vi "Update State.vi"(8 "error in (no error)":errorcluster, 11 "MF3 in":refnum<class "MF3.lvclass">) -> (0 "error out":errorcluster, 2 "fail?":bool, 3 "MF3 out":refnum<class "MF3.lvclass">)   [LabVIEW 2011, in "MF3.lvclass"]
uses:
  MF3.lvclass
  Controls/Motor Names.ctl
  MF3.lvclass/MF3.ctl
  <vilib>/Utility/error.llb/Error Cluster From Error Code.vi
  <vilib>/rvi/errors/niLvFpgaAdjustHostInterfaceError.vi
  <vilib>/rvi/interface/nirviReadWriteControl/nirviReadWriteControl.xnode
  FPGA Bitfiles/MotorsInterface.lvbitx
  NiFpgaLv.dll
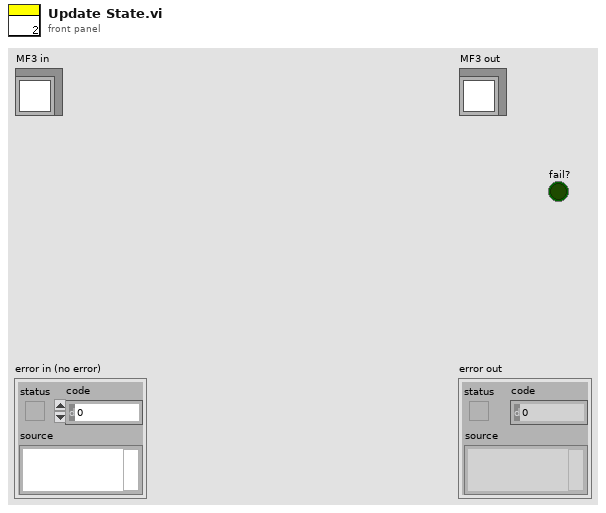
[diagram p1: front panel]
types:
  T1 = typedef "Motor Names.ctl" = enum16{"Thumb1", "Thumb2", "Thumb3", "Middle1", "Middle2", "Middle3", "Redundant", "Index1", "Index2", "Index3"}
  T2 = cluster{"Proportional Gain":i16, "Integral Gain":i16, "Derivative Gain":i16}
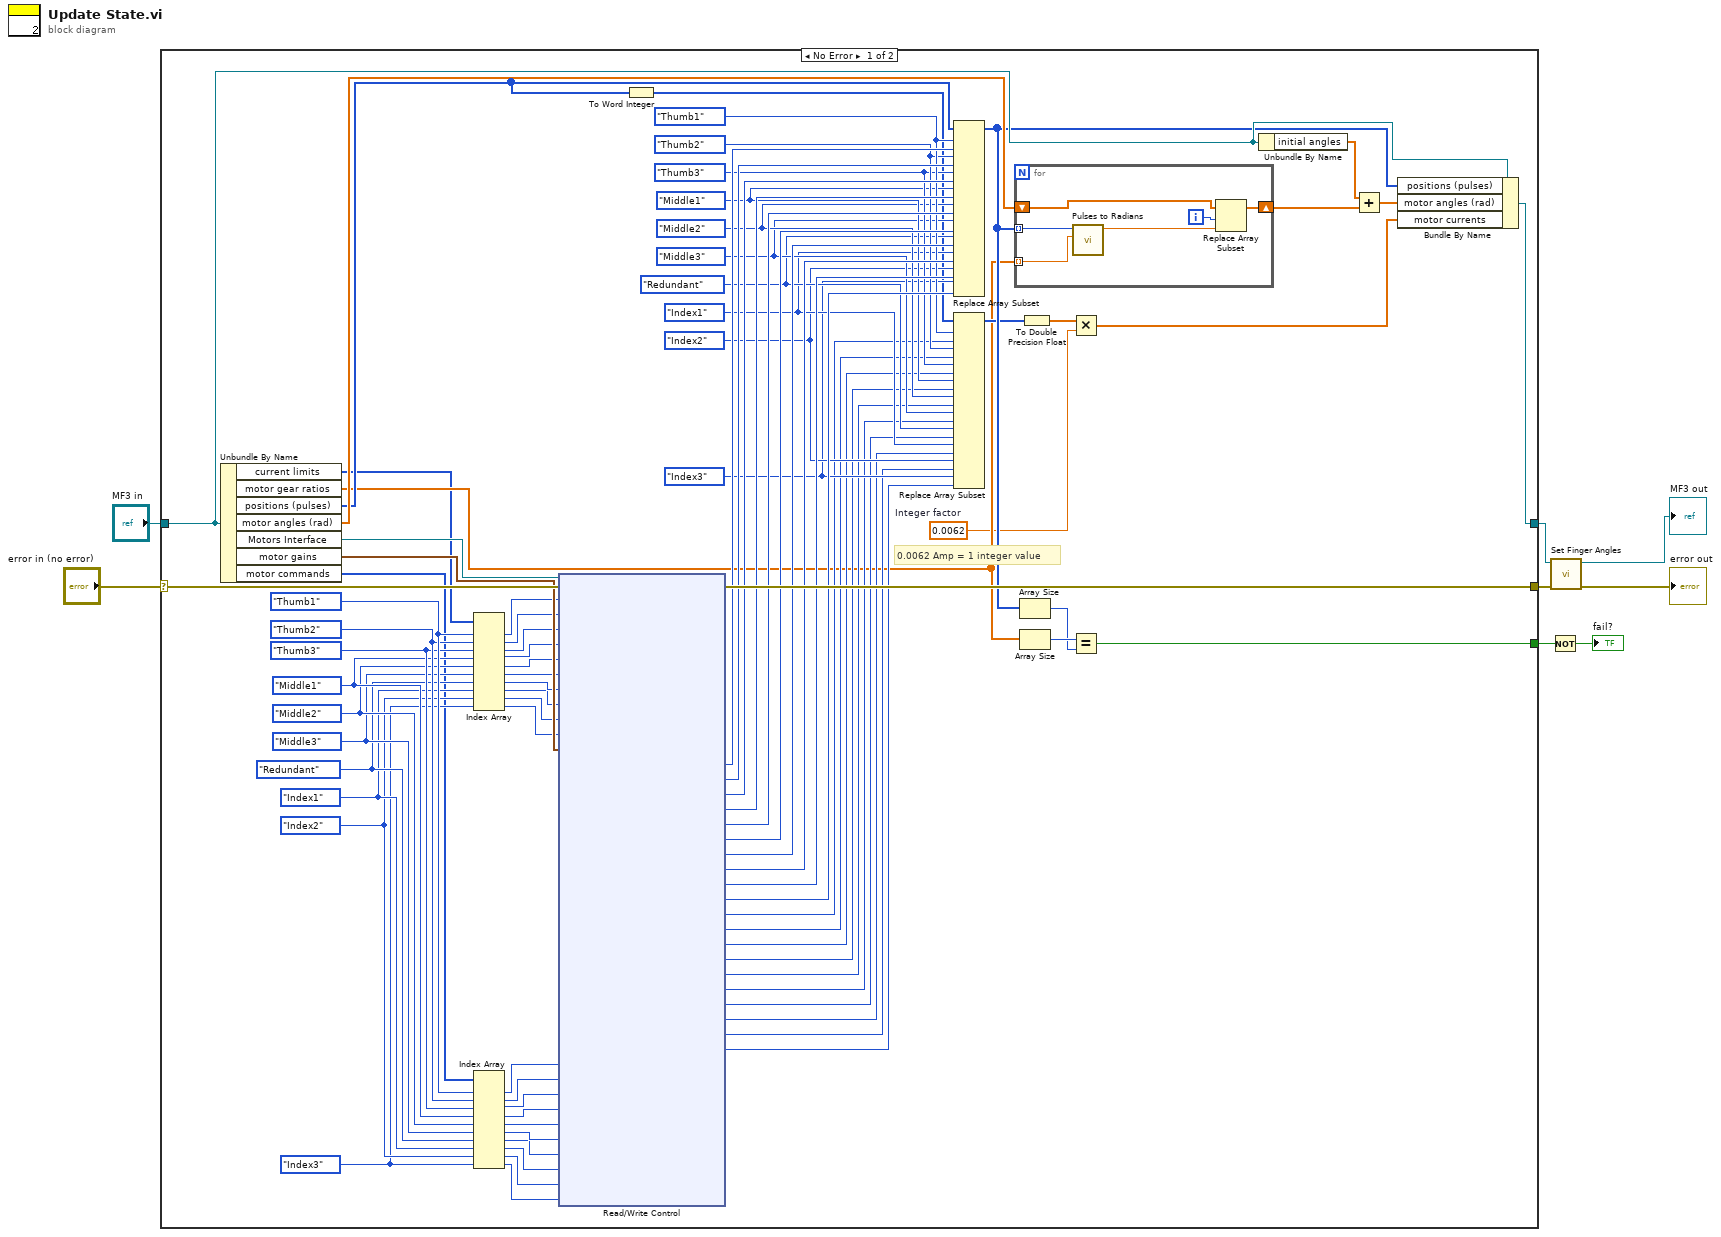
[diagram p0: block diagram]
diagram:
  n1 = case shown="No Error" "error in (no error)" {
    selector: "error in (no error)" -> [w90 w99]
    tunnel: [w89 w99] -> w3
    tunnel: [w88 w98] -> w4
    tunnel: "MF3 in" -> [w84 w98]
    tunnel: [w87 _] -> w6
    frame No Error {
      w29 = Motor_Names."Thumb1" ("Motor Names")
      w20 = Motor_Names."Index3" ("Motor Names")
      w21 = Motor_Names."Index2" ("Motor Names")
      w22 = Motor_Names."Index1" ("Motor Names")
      w23 = Motor_Names."Redundant" ("Motor Names")
      w24 = Motor_Names."Middle3" ("Motor Names")
      w25 = Motor_Names."Middle2" ("Motor Names")
      w26 = Motor_Names."Middle1" ("Motor Names")
      w27 = Motor_Names."Thumb3" ("Motor Names")
      w28 = Motor_Names."Thumb2" ("Motor Names")
      w42 = 0.0062  # Integer factor
      w61 = Motor_Names."Index3" ("Motor Names")
      w62 = Motor_Names."Index2" ("Motor Names")
      w63 = Motor_Names."Index1" ("Motor Names")
      w64 = Motor_Names."Redundant" ("Motor Names")
      w65 = Motor_Names."Middle3" ("Motor Names")
      w66 = Motor_Names."Middle2" ("Motor Names")
      w67 = Motor_Names."Middle1" ("Motor Names")
      w68 = Motor_Names."Thumb3" ("Motor Names")
      w69 = Motor_Names."Thumb2" ("Motor Names")
      w70 = Motor_Names."Thumb1" ("Motor Names")
      # "0.0062 Amp = 1 integer value"
      n2 = Unbundle By Name(w84) -> ("current limits"=w40:i16[], "motor gear ratios"=w45:dbl[], "positions (pulses)"=w57:i32[], "motor angles (rad)"=w86:dbl[], "Motors Interface"=w91:refnum<k20>, "motor gains"=w41:T2, "motor commands"=w19:i16[])
      n3 = Index Array(array=w40, index #1=w29, index #2=w28, index #3=w27, index #4=w26, index #5=w25, index #6=w24, index #7=w23, index #8=w22, index #9=w21, index #10=w20) -> (element #1=w39:i16, element #2=w37:i16, element #3=w36:i16, element #4=w35:i16, element #5=w34:i16, element #6=w33:i16, element #7=w32:i16, element #8=w31:i16, element #9=w30:i16, element #10=w38:i16)
      n4 = Index Array(array=w19, index #1=w29, index #2=w28, index #3=w27, index #4=w26, index #5=w25, index #6=w24, index #7=w23, index #8=w22, index #9=w21, index #10=w20) -> (element #1=w18:i16, element #2=w17:i16, element #3=w16:i16, element #4=w15:i16, element #5=w14:i16, element #6=w13:i16, element #7=w12:i16, element #8=w11:i16, element #9=w10:i16, element #10=w9:i16)
      n5 = xnode "Read/Write Control"("FPGA VI Reference In"=w91, "error in"=w90, "Current Limit Thumb 1"=w39, "Current Limit Thumb 2"=w37, "Current Limit Thumb 3"=w36, "Current Limit Middle 1"=w35, "Current Limit Middle 2"=w34, "Current Limit Middle 3"=w33, "Current Limit Redundant"=w32, "Current Limit Index 1"=w31, "Current Limit Index 2"=w30, "Current Limit Index 3"=w38, "Motors Gains"=w41, "Current Setpoint Thumb 1"=w18, "Current Setpoint Thumb 2"=w17, "Current Setpoint Thumb 3"=w16, "Current Setpoint Middle 1"=w15, "Current Setpoint Middle 2"=w14, "Current Setpoint Middle 3"=w13, "Current Setpoint Redundant"=w12, "Current Setpoint Index 1"=w11, "Current Setpoint Index 2"=w10, "Current Setpoint Index 3"=w9) -> ("error out"=w89:errorcluster, "Position Thumb 1"=w80:i32, "Position Thumb 2"=w79:i32, "Position Thumb 3"=w78:i32, "Position Middle 1"=w77:i32, "Position Middle 2"=w76:i32, "Position Middle 3"=w75:i32, "Position Redundant"=w74:i32, "Position Index 1"=w73:i32, "Position Index 2"=w72:i32, "Position Index 3"=w71:i32, "Current Thumb 1"=w58:i16, "Current Thumb 2"=w55:i16, "Current Thumb 3"=w54:i16, "Current Middle 1"=w53:i16, "Current Middle 2"=w52:i16, "Current Middle 3"=w51:i16, "Current Redundant"=w50:i16, "Current Index 1"=w49:i16, "Current Index 2"=w48:i16, "Current Index 3"=w47:i16)  [unwired: 1 out]
      n6 = To Word Integer(number=w57) -> (16bit integer=w56:i16[])
      n7 = Replace Array Subset(array=w57, new element #1=w80, index #1=w70, new element #2=w79, index #2=w69, new element #3=w78, index #3=w68, new element #4=w77, index #4=w67, new element #5=w76, index #5=w66, new element #6=w75, index #6=w65, new element #7=w74, index #7=w64, new element #8=w73, index #8=w63, new element #9=w72, index #9=w62, new element #10=w71, index #10=w61) -> (w60:i32[])
      n8 = Replace Array Subset(array=w56, new element #1=w58, index #1=w70, new element #2=w55, index #2=w69, new element #3=w54, index #3=w68, new element #4=w53, index #4=w67, new element #5=w52, index #5=w66, new element #6=w51, index #6=w65, new element #7=w50, index #7=w64, new element #8=w49, index #8=w63, new element #9=w48, index #9=w62, new element #10=w47, index #10=w61) -> (w59:i16[])
      n9 = for {
        shift-right: [w94] -> w85
        shift-left: w86 -> [w97]
        tunnel: w60 -> [w93] mode=indexing
        tunnel: w45 -> [w92] mode=indexing
        i -> [w96]
        n10 = call "Pulses to Radians.vi"("gear ratio"=w92, "encoder pulses"=w93) -> ("angle (rad)"=w95:dbl)  [unwired: 9 in]
        n11 = Replace Array Subset(array=w97, new element=w95, index=w96) -> (w94:dbl[])
      }
      n12 = Array Size(array=w60) -> (size(s)=w81:i32)
      n13 = Array Size(array=w45) -> (size(s)=w82:i32)
      n14 = To Double Precision Float(number=w59) -> (double precision float=w46:dbl[])
      n15 = Multiply(x=w46, y=w42) -> (x*y=w43:dbl[])
      n16 = Equal?(x=w82, y=w81) -> (x = y?=w87:bool)
      n17 = Unbundle By Name(w84) -> ("initial angles"=w83:dbl[])
      n18 = Add(x=w83, y=w85) -> (x+y=w44:dbl[])
      n19 = Bundle By Name(cluster=w84, "positions (pulses)"=w60, "motor angles (rad)"=w44, "motor currents"=w43) -> (w88:refnum<class "MF3.lvclass">)
    }
    frame Error {
    }
  }
  n20 = Not(x=w6) -> (.not. x?=→"fail?":bool)
  n21 = call "Set Finger Angles.vi"("error in (no error)"=w3, "MF3 in"=w4) -> ("error out"=→"error out":errorcluster, "MF3 out"=→"MF3 out":refnum<class "MF3.lvclass">)  [unwired: 8 in]
